vi "Frame Calc Add.vi"(4 "Array Position":i32, 5 "Tlg Data Array In":T2 {"CAN frame In"."FlexRay"."cycle count" max=63 step=1; "CAN frame In"."payload" format="%x"; "CAN frame In"."identifier / slot" format="%x"; "FlexRay Channel" items=["A", "B", "A+B"]}, 7 "Frame In":T1={"timestamp"=timestamp(0 s since 1904-01-01), "payload"=[0, 0, 0, 0, 0, 0, 0, 0], "identifier / slot"=0, "Data type"=0, "payload length"=0, "CAN"={"extended?"=FALSE}, "FlexRay"={"cycle count"=0, "startup?"=FALSE, "sync?"=FALSE, "preamble?"=FALSE, "ch A"=FALSE, "ch B"=FALSE, "macrotick"=32}, "echo?"=FALSE} {"FlexRay"."cycle count" max=63 step=1; "payload" format="%x"; "identifier / slot" format="%x"}) -> (1 "Tlg Data Array Out":T2 {"CAN frame In"."FlexRay"."cycle count" max=63 step=1; "CAN frame In"."payload" format="%x"; "CAN frame In"."identifier / slot" format="%x"; "FlexRay Channel" items=["A", "B", "A+B"]}, 3 "Frame Out":T1={"timestamp"=timestamp(0 s since 1904-01-01), "payload"=[0, 0, 0, 0, 0, 0, 0, 0], "identifier / slot"=0, "Data type"=0, "payload length"=0, "CAN"={"extended?"=FALSE}, "FlexRay"={"cycle count"=0, "startup?"=FALSE, "sync?"=FALSE, "preamble?"=FALSE, "ch A"=FALSE, "ch B"=FALSE, "macrotick"=32}, "echo?"=FALSE} {"FlexRay"."cycle count" max=63 step=1; "payload" format="%x"; "identifier / slot" format="%x"})   [LabVIEW 2014, in "CAN Bus Monitor Engine.lvlib"]
uses:
  CAN Bus Monitor Engine.lvlib
  Controls/Analyze Array.ctl
  Controls/FlexRay Channel.ctl
  Controls/XNET BM Frame.ctl
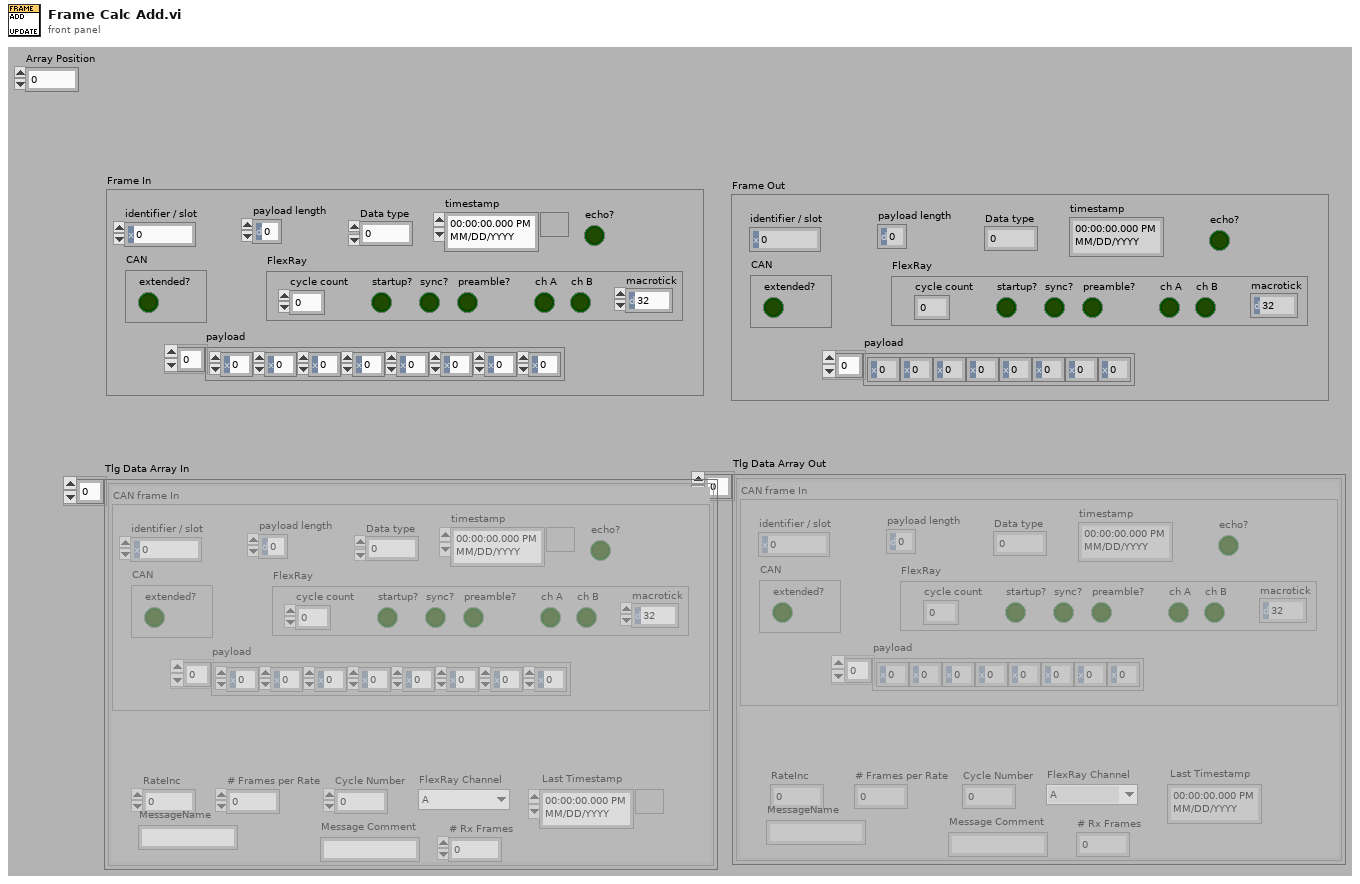
[diagram p1: front panel]
types:
  T1 = typedef "CAN Bus Monitor Engine.lvlib/XNET BM Frame.ctl" = cluster{"timestamp":timestamp, "payload":u8[], "identifier / slot":u32, "Data type":u8, "payload length":u8, "CAN":cluster{"extended?":bool}, "FlexRay":cluster{"cycle count":u8, "startup?":bool, "sync?":bool, "preamble?":bool, "ch A":bool, "ch B":bool, "macrotick":u16}, "echo?":bool}
  T2 = typedef "CAN Bus Monitor Engine.lvlib/Analyze Array.ctl" = cluster{"# Rx Frames":u32, "Last Timestamp":timestamp, "RateInc":dbl, "# Frames per Rate":u32, "MessageName":string, "Cycle Number":u32, "FlexRay Channel":T3, "Message Comment":string, "CAN frame In":T1}[]
  T3 = typedef "CAN Bus Monitor Engine.lvlib/FlexRay Channel.ctl" = u16
  T4 = cluster{"# Rx Frames":u32, "Last Timestamp":timestamp, "RateInc":dbl, "# Frames per Rate":u32, "MessageName":string, "Cycle Number":u32, "FlexRay Channel":T3, "Message Comment":string, "CAN frame In":T1}
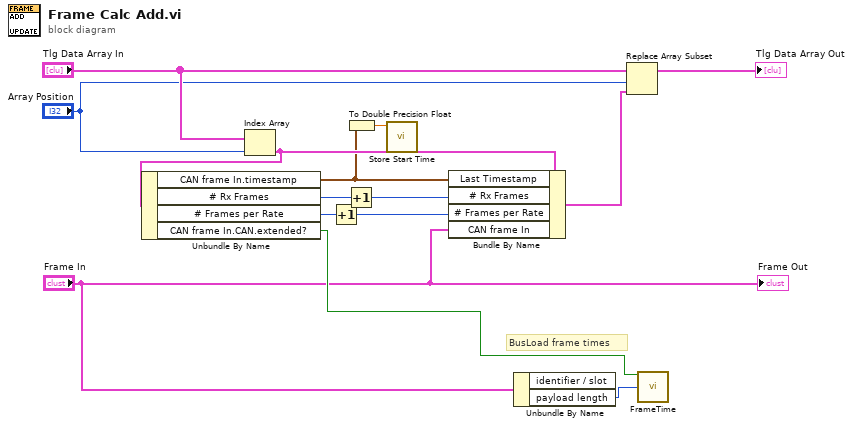
[diagram p0: block diagram]
diagram:
  # "BusLoad frame times"
  n1 = Index Array(array="Tlg Data Array In", index="Array Position") -> (element=w10:T4)
  n2 = Unbundle By Name(w10) -> ("CAN frame In.timestamp"=w3:timestamp, "# Rx Frames"=w9:u32, "# Frames per Rate"=w7:u32, "CAN frame In.CAN.extended?"=w5:bool)
  n3 = Increment(x=w7) -> (x+1=w6:u32)
  n4 = Increment(x=w9) -> (x+1=w8:u32)
  n5 = To Double Precision Float(number=w3) -> (double precision float=w4:dbl)
  n6 = call "Store Start Time.vi"("Timestamp"=w4) -> ()  [unwired: 11 in]
  n7 = Bundle By Name(cluster=w10, "Last Timestamp"=w3, "# Rx Frames"=w8, "# Frames per Rate"=w6, "CAN frame In"="Frame In") -> (w11:T4)
  n8 = Unbundle By Name("Frame In") -> ("payload length"=w1:u8)  [unwired: 1 out]
  n9 = Replace Array Subset(array="Tlg Data Array In", new element=w11, index="Array Position") -> (→"Tlg Data Array Out":T2)
  n10 = call "FrameTime.vi"("Is Extended ID?"=w5, "DataLength"=w1) -> ()  [unwired: 14 in]
  "Frame Out" <- "Frame In"
